vi "2D-LIF_CDN.vi"() -> ()   [LabVIEW 2022 SP3]
uses:
  dyelaser.lib/Sirah Control API.llb/SC API Burst Scan Mode.ctl
panel:
  out "Final.Gate.Delay":u64=600
  in  "New Scan":bool
  in  "Shut Down":bool
  out "ScanWhat?":enum16{"Nothing", "Lumonics", "Delay"}(ring)
  in  "Pause Scan":bool
  in  "Live Monitor":bool
  in  "force continue":bool
  in  "Force stop":bool
  out "State":T1(ring)=enum."Wait for input"
  in  "Abort Scan":bool
  in  "Camera":T2={"Gate.Delay"=0, "Delay.Step"=0, "Gate.Duration"=50, "#Accum"=30, "SetpointTemp"=-30, "Last Temp"=0, "Current Temp"=0}
  out "Data":cluster{"CCD":i32[], "2D LIF data":i32[][]}
  in  "Mono":T3={"Offset (cm-1)"=200.0, "Step (cm-1)"=2.0, "Counter"=165.13, "Scan Step/Mono Step"=1, "Status"={"Moving"=FALSE, "Home"=FALSE, "Hi"=FALSE, "Low"=FALSE}, "nm"=660.502, "Mono port"="McPherson"} {"nm" format="%.3f"; "Scan Step/Mono Step" format="%.2f"; "Counter" format="%.2g"; "Step (cm-1)" format="%.1f"; "Offset (cm-1)" format="%#.4g"}
  in  "DyeLaser":T4={"Scan.Start (cm-1)"=15340.0, "Scan.Stop (cm-1)"=15365.0, "Scan.step (cm-1)"=0.05, "Dye laser port"="USB0::0x17E7::0x0500::11-20-16::INSTR", "Laser"=enum."Hyperdye", "NPoints"=501, "CurrentStep"=0, "Current.cm-1"=15340.0} {"Current.cm-1" format="%.2f"; "Scan.Stop (cm-1)" format="%.2f"; "Scan.step (cm-1)" format="%.2g"; "Scan.Start (cm-1)" format="%.2f"}
  # "ns"
  # "ns"
  # "ns"
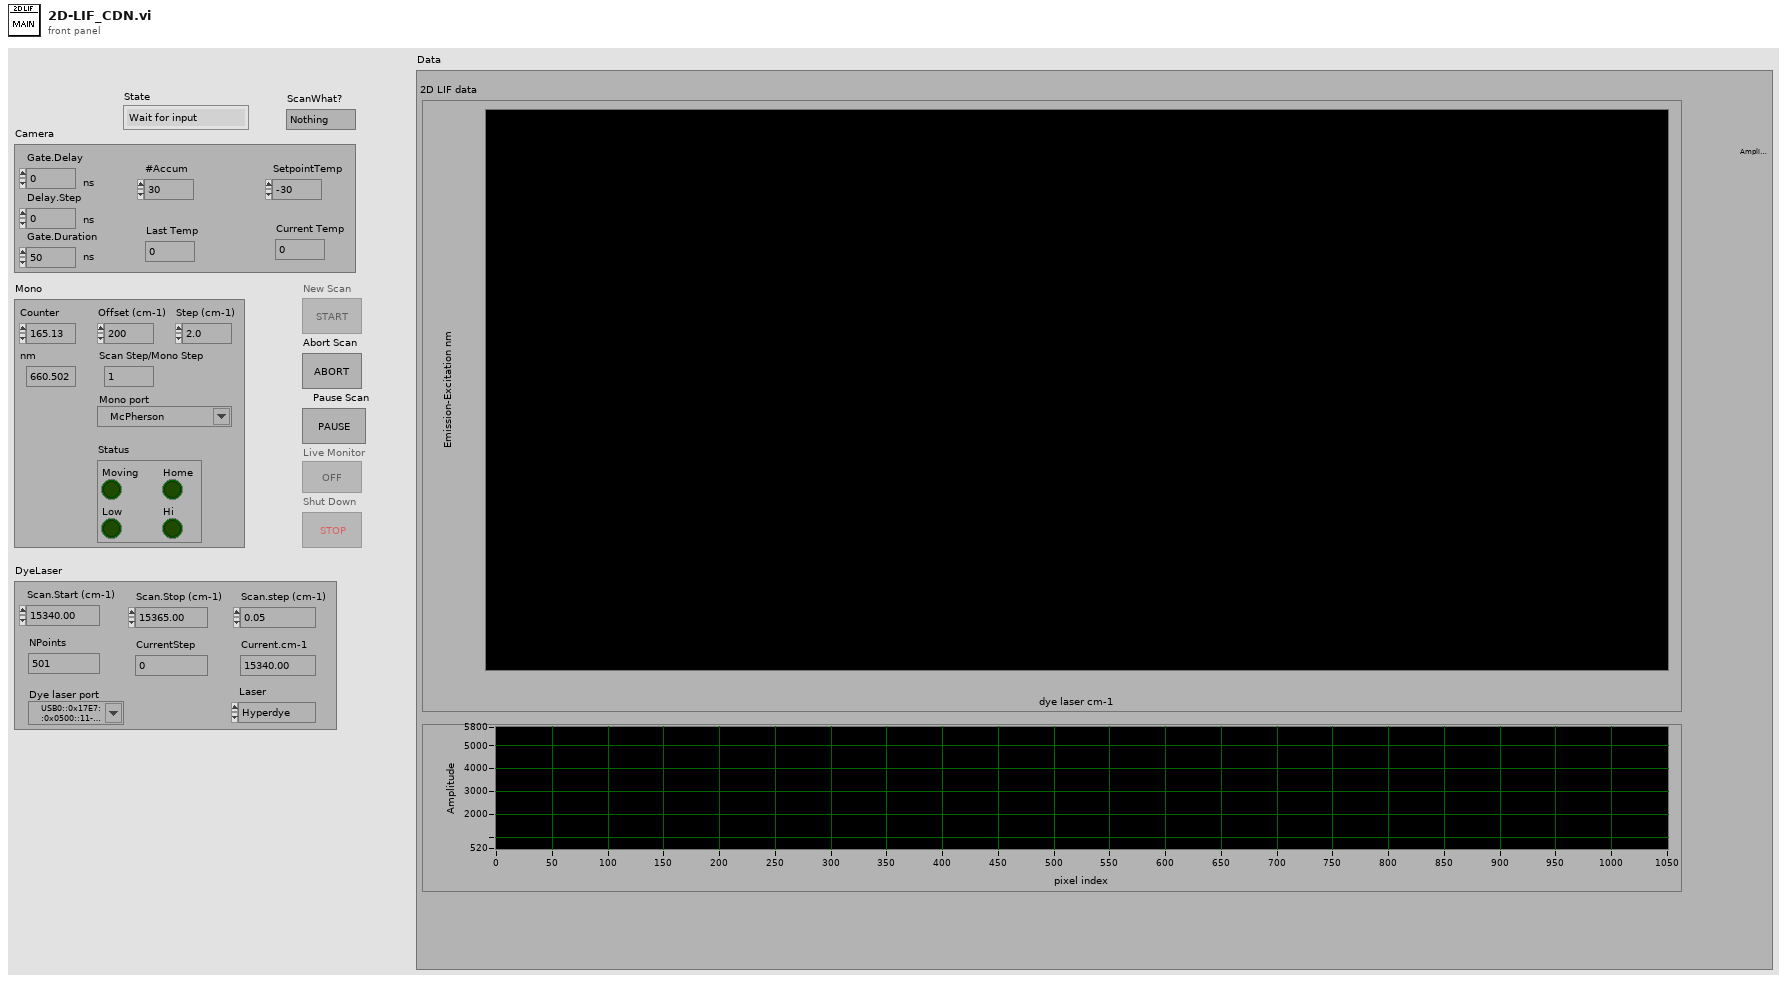
[diagram p1: front panel]
types:
  T1 = enum16{"Connect", "Wait for input", "Initialize", "Live", "Start Scan", "Continue Scan", "End Scan", "Shut Down"}
  T2 = cluster{"Gate.Delay":u64, "Delay.Step":u64, "Gate.Duration":u64, "#Accum":i32, "SetpointTemp":i32, "Last Temp":i32, "Current Temp":i32}
  T3 = cluster{"Offset (cm-1)":dbl, "Step (cm-1)":dbl, "Counter":dbl, "Scan Step/Mono Step":i32, "Status":cluster{"Moving":bool, "Home":bool, "Hi":bool, "Low":bool}, "nm":dbl, "Mono port":refnum<visa-resource-name>}
  T4 = cluster{"Scan.Start (cm-1)":dbl, "Scan.Stop (cm-1)":dbl, "Scan.step (cm-1)":dbl, "Dye laser port":refnum<visa-resource-name>, "Laser":enum16{"Syrah", "Hyperdye"}, "NPoints":i32, "CurrentStep":i32, "Current.cm-1":dbl}
  T5 = typedef "SC API Burst Scan Mode.ctl" = enum16{"Wavelength (nm), use increment", "Wavenumber (cm-1), use increment", "Frequency (Hz), use increment", "x", "xx", "xxx", "xxxx", "xxxxx", "xxxxxx", "xxxxxxx", "Wavelength (nm), use number", "Wavenumber (cm-1), use number", "Frequency (Hz), use number"}
  T6 = enum8{"Enabled", "Disabled", "Disabled and Grayed Out"}
  T7 = cluster{"offset (cm-1)":dbl, "step (cm-1)":dbl, "Counter":dbl, "Scanstep/monostep":i32, "Status":cluster{"Moving":bool, "Home":bool, "Hi":bool, "Low":bool}, "nm":dbl, "mono port":refnum<visa-resource-name>}
  T8 = cluster{"Scan.Start (cm-1)":dbl, "Scan.Stop (cm-1)":dbl, "Scan.step (cm-1)":dbl, "dye laser port":refnum<visa-resource-name>, "Laser":enum16{"Syrah", "Hyperdye"}, "NSteps":i32, "CurrentStep":i32, "Current.cm-1":dbl}
  T9 = cluster{"offset (cm-1)":dbl, "step (cm-1)":dbl, "Counter":dbl, "Scanstep/monostep":i32, "Status":cluster{"Moving":bool, "Home":bool, "Hi":bool, "Low":bool}, "nm":dbl, "Mono port":refnum<visa-resource-name>}
  T10 = cluster{"Scan.Start (cm-1)":dbl, "Scan.Stop (cm-1)":dbl, "Scan.step (cm-1)":dbl, "dye laser port":refnum<visa-resource-name>, "Laser":enum16{"Syrah", "Hyperdye"}, "NPoints":i32, "CurrentStep":i32, "Current.cm-1":dbl}
  T11 = cluster{"offset (cm-1)":dbl, "step (cm-1)":dbl, "Counter":dbl, "Scanstep/monostep":i32, "Status":cluster{"Moving":bool, "Home":bool, "Hi":bool, "Low":bool}, "nm":dbl, "VISA resource name":refnum<visa-resource-name>}
  T12 = cluster{"Scan.Start (cm-1)":dbl, "Scan.Stop (cm-1)":dbl, "Scan.step (cm-1)":dbl, "VISA resource name":refnum<visa-resource-name>, "Laser":enum16{"Syrah", "Hyperdye"}, "NSteps":i32, "CurrentStep":i32, "Current.cm-1":dbl}
  T13 = cluster{"Scan.Start (cm-1)":dbl, "Scan.Stop (cm-1)":dbl, "Scan.step (cm-1)":dbl, "Dye laser port":refnum<visa-resource-name>, "Laser":enum16{"Syrah", "Hyperdye"}, "NSteps":i32, "CurrentStep":i32, "Current.cm-1":dbl}
  T14 = typedef "LVRangeTypeDef.ctl" = cluster{"Minimum":dbl, "Maximum":dbl, "Increment":dbl, "Minor Increment":dbl, "Start":dbl}
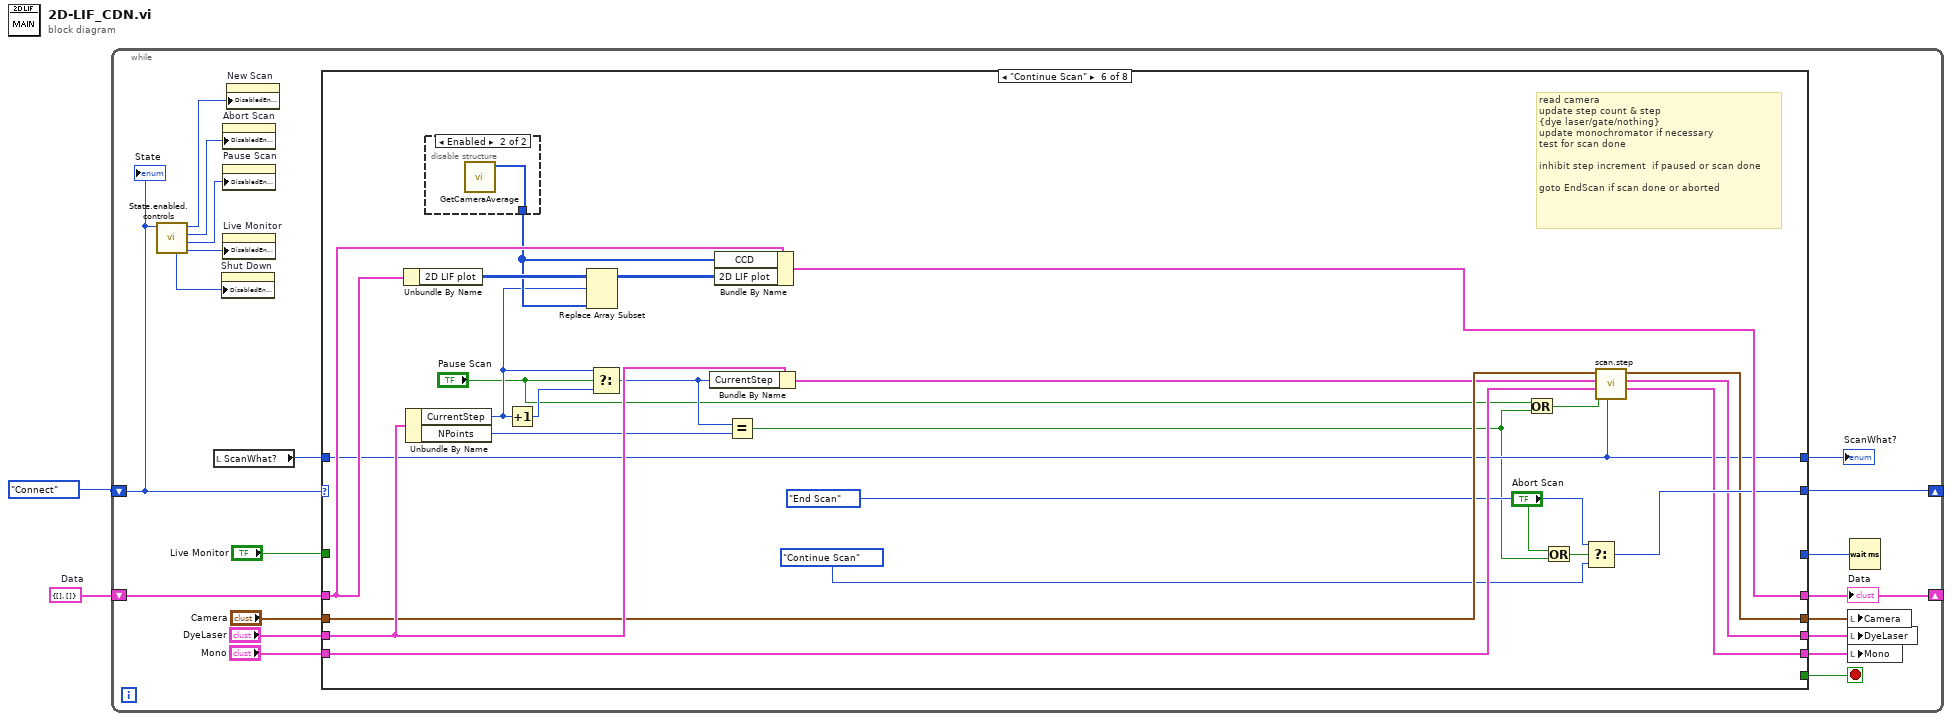
[diagram p0: block diagram]
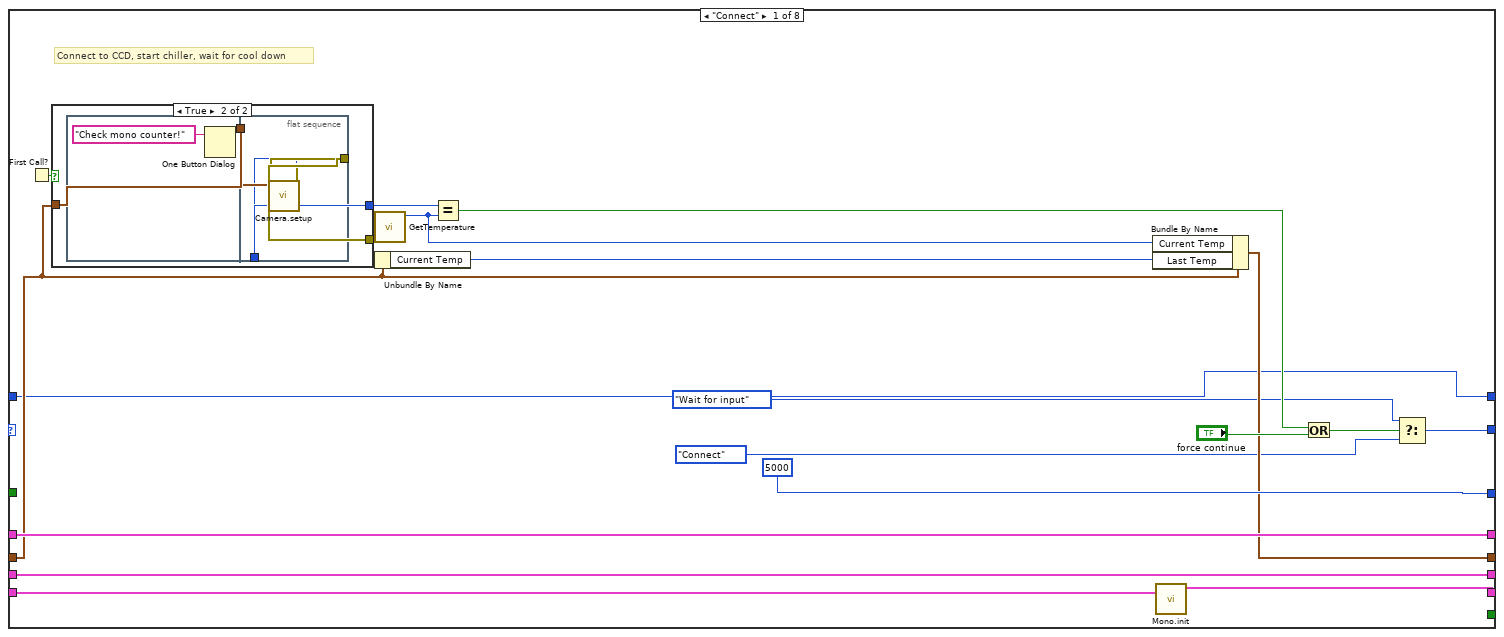
[diagram p2: hidden frame]
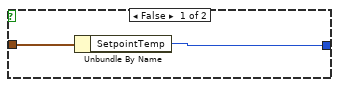
[diagram p3: hidden frame]
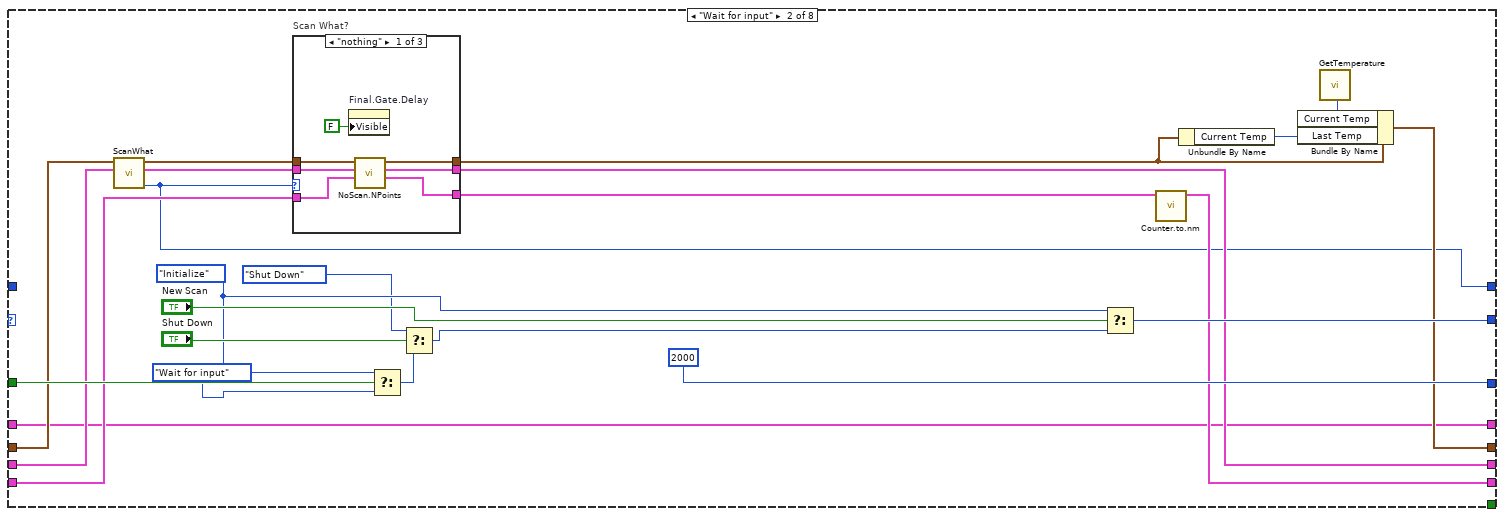
[diagram p4: hidden frame]
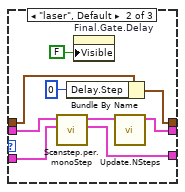
[diagram p5: hidden frame]
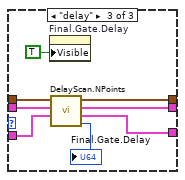
[diagram p6: hidden frame]
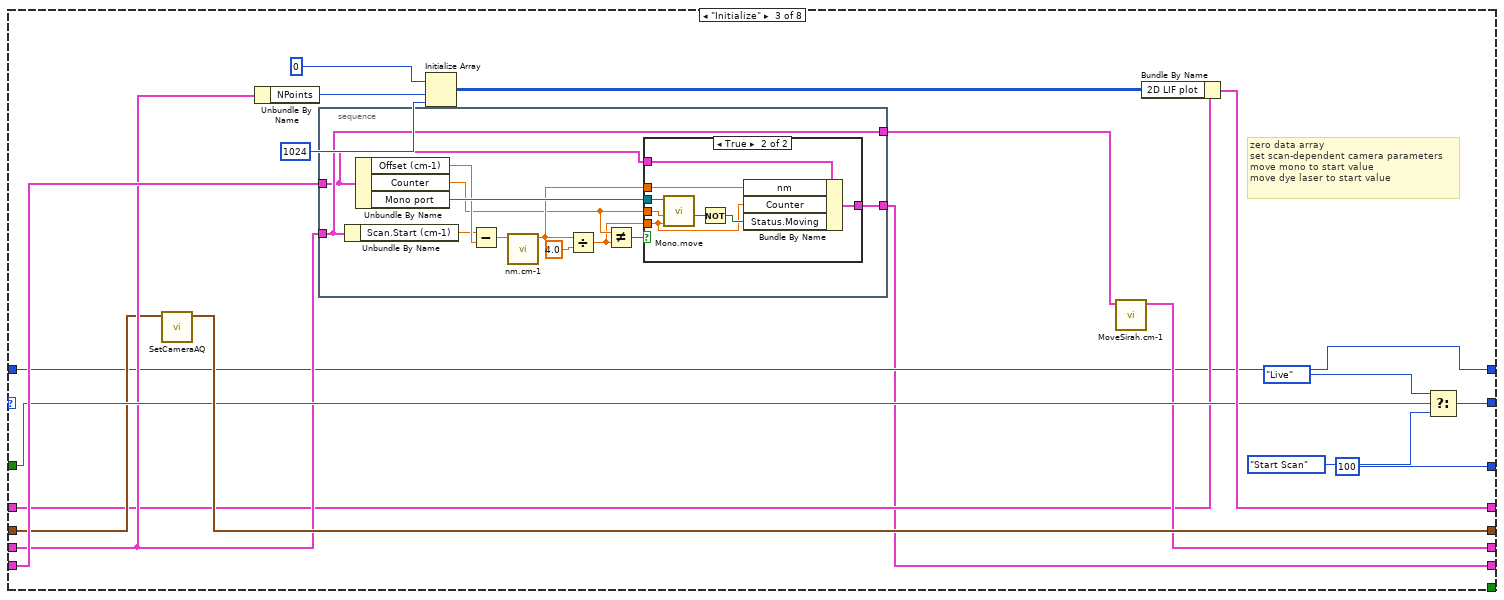
[diagram p7: hidden frame]
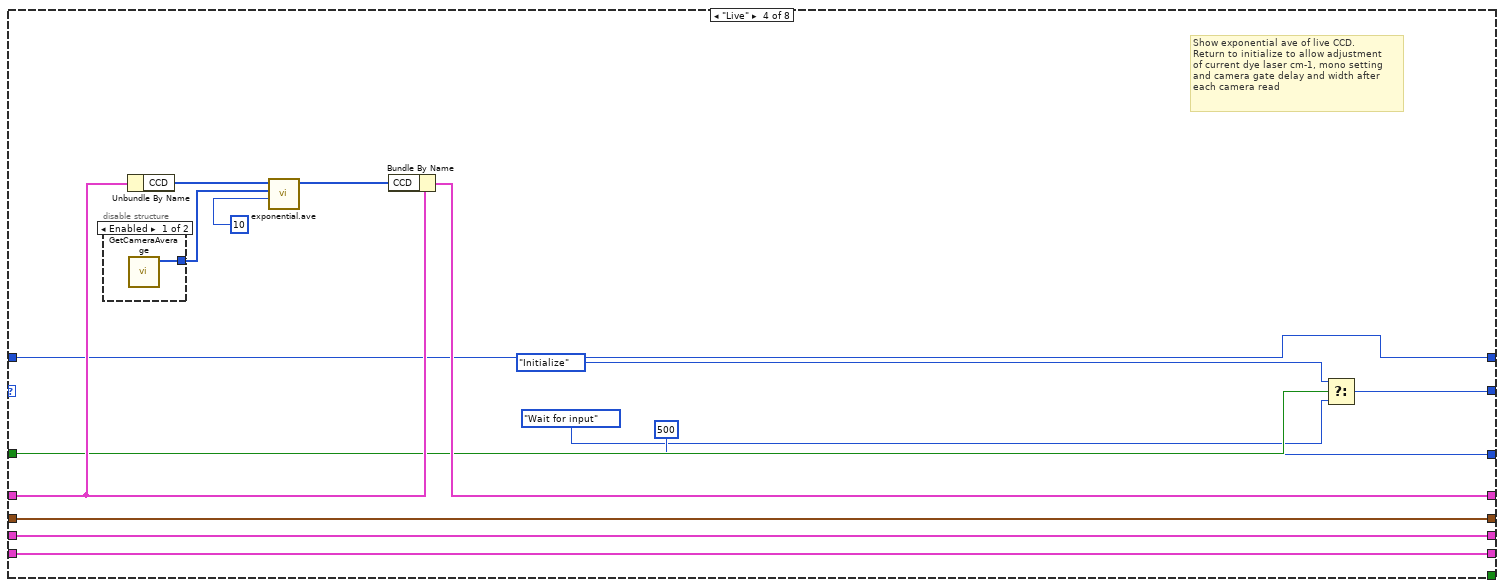
[diagram p9: hidden frame]
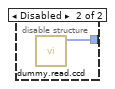
[diagram p10: hidden frame]
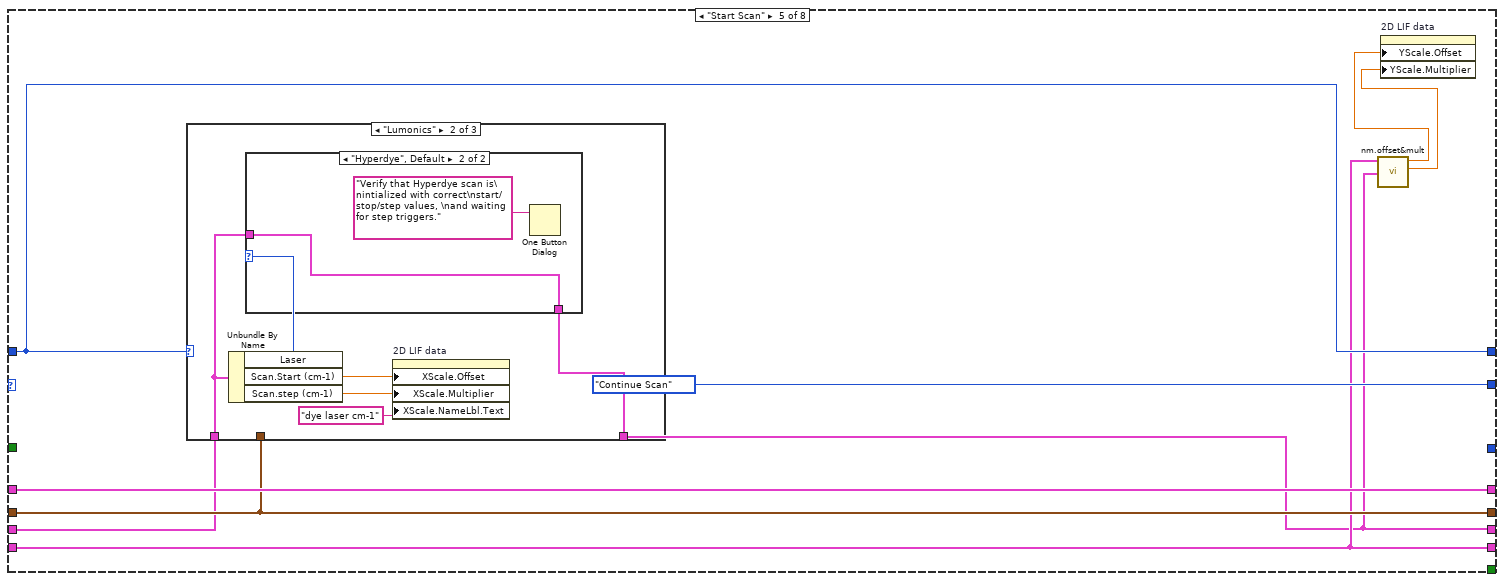
[diagram p11: hidden frame]
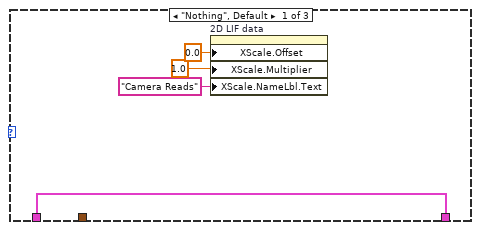
[diagram p12: hidden frame]
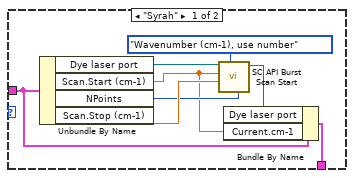
[diagram p13: hidden frame]
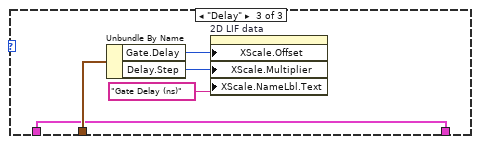
[diagram p14: hidden frame]
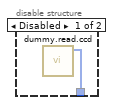
[diagram p15: hidden frame]
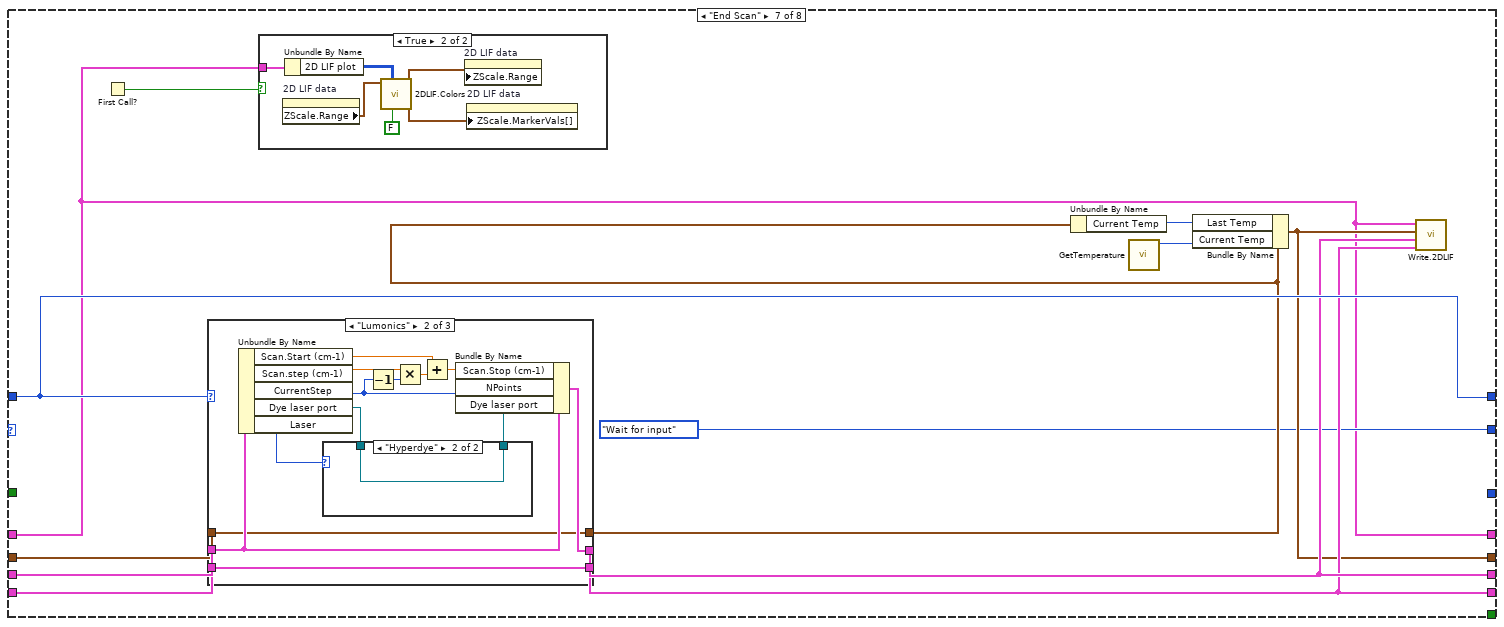
[diagram p16: hidden frame]
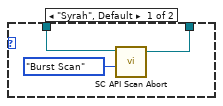
[diagram p19: hidden frame]
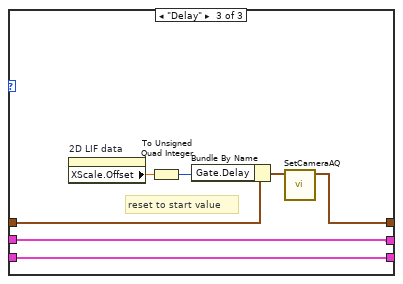
[diagram p20: hidden frame]
diagram:
  w2 = cluster{"CCD":i32[], "2D LIF plot":i32[][]} {"CCD"=[], "2D LIF plot"=[]}  # Data
  n1 = while {
    shift-right: [w20] -> _
    shift-left: w2 -> [w21]
    shift-right: [w6] -> _
    shift-left: T1."Connect" ("State") -> [w3]
    stop <- w22 stop-if-true
    n2 = call "State.enabled.controls.vi"("state"=w3) -> ("live"=w12:T6, "pause"=w11:T6, "abort"=w10:T6, "start"=w5:T6, "stop"=w4:T6)  [unwired: 6 in]
    n3 = local read "ScanWhat?"() -> (w9:enum16{"Nothing", "Lumonics", "Delay"})
    n4 = property on="Shut Down" class="Bool"("DisabledEnum"=w4) -> ()  [unwired: 2 in, 2 out]
    n5 = property on="Abort Scan" class="Bool"("DisabledEnum"=w10) -> ()  [unwired: 2 in, 2 out]
    n6 = property on="Pause Scan" class="Bool (strict)"("DisabledEnum"=w11) -> ()  [unwired: 2 in, 2 out]
    n7 = property on="Live Monitor" class="Bool (strict)"("DisabledEnum"=w12) -> ()  [unwired: 2 in, 2 out]
    n8 = property on="New Scan" class="Bool"("DisabledEnum"=w5) -> ()  [unwired: 2 in, 2 out]
    n9 = case shown="\"Continue Scan\"" w3 {
      tunnel: [_ _ _ _ _ _ _ w265] -> w22
      tunnel: w21 -> [w41 w52 w104 w152 w164 w214 w218 w274]
      tunnel: [w41 w52 w115 w150 w164 w209 w218 w274] -> w20
      tunnel: [w31 w56 w107 w147 w158 w201 w226 w267] -> w19
      tunnel: "Camera" -> [w26 w64 w105 w144 w163 w203 w222 w269]
      tunnel: [w32 w59 w112 w144 w163 w202 w220 w268] -> w13
      tunnel: "DyeLaser" -> [w31 w63 w106 w147 w162 w207 w225 w267]
      tunnel: "Mono" -> [w28 w65 w111 w151 w159 w198 w224 w270]
      tunnel: [u32 5000 u32 2000 ("milliseconds to wait") u32 100 ("milliseconds to wait") u32 500 ("milliseconds to wait") _ _ _ u32 5000] -> w16
      tunnel: [w27 w57 w99 w151 w159 w200 w223 w270] -> w15
      tunnel: [w29 w70 w110 w153 T1."Continue Scan" ("State") w206 T1."Wait for input" ("State") T1."Shut Down" ("State")] -> w6
      tunnel: "Live Monitor" -> [_ w68 w109 w148 _ _ _ _]
      tunnel: [w25 w51 w103 w142 w160 w197 w227 w264] -> w8
      tunnel: w9 -> [w25 _ w103 w142 w160 w197 w227 w264]
      frame "Connect" {
        # "Connect to CCD, start chiller, wait for cool down"
        n10 = First Call?() -> (First Call?: T/F=w40:bool)
        n11 = case shown="True" w40 {
          tunnel: [_ w45] -> w39
          tunnel: [w43 w44] -> w38
          tunnel: w26 -> [w42 w46]
          frame False {
            n12 = Unbundle By Name(w42) -> ("SetpointTemp"=w43:i32)
          }
          frame True {
            n13 = flat-sequence {
              tunnel: w46 -> [w50]
              tunnel: [w49] -> w45
              tunnel: [w48] -> w44
              frame #0 {
                n14 = One Button Dialog(message="Check mono counter!") -> ()  [unwired: 1 in, 1 out]
              }
              frame #1 {
                n15 = call "Camera.setup.vi"("Camera"=w50) -> ("error out"=w49:errorcluster, "SetpointTemp"=w48:i32)  [unwired: 8 in, 1 out]
              }
            }
          }
        }
        n16 = call "GetTemperature.vi"("error in (no error)"=w39) -> ("temperature"=w37:i32)  [unwired: 3 in, 3 out]
        n17 = Unbundle By Name(w26) -> ("Current Temp"=w30:i32)
        n18 = Equal?(x=w38, y=w37) -> (x = y?=w34:bool)
        n19 = Bundle By Name(cluster=w26, "Current Temp"=w37, "Last Temp"=w30) -> (w32:T2)
        n20 = call "Mono.init.vi"("Mono in"=w28) -> ("Mono out"=w27:T7)  [unwired: 10 in]
        n21 = Or(x=w34, y="force continue") -> (x .or. y?=w36:bool)
        n22 = Select(t=T1."Wait for input" ("State"), s=w36, f=T1."Connect" ("State")) -> (s? t:f=w29:T1)
      }
      frame "Wait for input" {
        w54 = T1."Initialize" ("State")
        n23 = call "ScanWhat.vi"("DyeLaser"=w63, "Camera"=w64) -> ("ScanWhat?"=w51:enum16{"nothing", "laser", "delay"}, "DyeLaser out"=w61:T8, "Camera out"=w62:T2)  [unwired: 7 in]
        n24 = case "Scan What?" shown="\"nothing\"" w51 {
          tunnel: w61 -> [w80 w89 w98]
          tunnel: w62 -> [w81 w83 w94]
          tunnel: w65 -> [w79 w90 w97]
          tunnel: [w78 w84 w93] -> w60
          tunnel: [w77 w86 w96] -> w56
          tunnel: [w76 w88 w95] -> w58
          frame "nothing" {
            n25 = property on="Final.Gate.Delay" class="DigNum (strict)"("Visible"=FALSE) -> ()  [unwired: 2 in, 2 out]
            n26 = call "NoScan.NPoints.vi"("Mono"=w79, "DyeLaser In"=w80, "Camera"=w81) -> ("Mono out"=w76:T9, "DyeLaser out"=w77:T10, "Camera out"=w78:T2)  [unwired: 6 in]
          }
          frame "laser", Default {
            n27 = call "Scanstep.per.monoStep.vi"("Mono in"=w90, "DyeLaser"=w89) -> ("Mono out"=w88:T11, "DyeLaser out"=w87:T12)  [unwired: 8 in]
            n28 = Bundle By Name(cluster=w83, "Delay.Step"=u64 0) -> (w84:T2)
            n29 = property on="Final.Gate.Delay" class="DigNum (strict)"("Visible"=FALSE) -> ()  [unwired: 2 in, 2 out]
            n30 = call "Update.NSteps.vi"("DyeLaser In"=w87) -> ("DyeLaser out"=w86:T10)  [unwired: 10 in]
          }
          frame "delay" {
            n31 = property on="Final.Gate.Delay" class="DigNum (strict)"("Visible"=TRUE) -> ()  [unwired: 2 in, 2 out]
            n32 = call "DelayScan.NPoints.vi"("Mono"=w97, "DyeLaser In"=w98, "Camera"=w94) -> ("Final.Gate.Delay"=→"Final.Gate.Delay":u64, "Mono out"=w95:T9, "DyeLaser out"=w96:T10, "Camera out"=w93:T2)  [unwired: 5 in]
          }
        }
        n33 = Select(t=w54, s=w68, f=T1."Wait for input" ("State")) -> (s? t:f=w69:T1)
        n34 = Select(t=T1."Shut Down" ("State"), s="Shut Down", f=w69) -> (s? t:f=w72:T1)
        n35 = Select(t=w54, s="New Scan", f=w72) -> (s? t:f=w70:T1)
        n36 = call "Counter.to.nm.vi"("Mono in"=w58) -> ("Mono out"=w57:T11)  [unwired: 10 in]
        n37 = Unbundle By Name(w60) -> ("Current Temp"=w66:i32)
        n38 = call "GetTemperature.vi"() -> ("temperature"=w67:i32)  [unwired: 4 in, 3 out]
        n39 = Bundle By Name(cluster=w60, "Current Temp"=w67, "Last Temp"=w66) -> (w59:T2)
      }
      frame "Initialize" {
        # "zero data array\nset scan-dependent camera parameters\nmove mono to start value\nmove dye laser to start value"
        n40 = call "SetCameraAQ.vi"("Camera"=w105) -> ("Camera out"=w112:T2)  [unwired: 9 in, 1 out]
        n41 = Unbundle By Name(w106) -> ("NPoints"=w113:i32)
        n42 = stacked-sequence {
          tunnel: w106 -> [w128]
          tunnel: [w128] -> w108
          tunnel: w111 -> [w127]
          tunnel: [w129] -> w99
          frame #0 {
            n43 = Unbundle By Name(w128) -> ("Scan.Start (cm-1)"=w124:dbl)
            n44 = Unbundle By Name(w127) -> ("Offset (cm-1)"=w125:dbl, "Counter"=w120:dbl, "Mono port"=w126:refnum<visa-resource-name>)
            n45 = Subtract(x=w124, y=w125) -> (x-y=w123:dbl)
            n46 = call "nm.cm-1.vi"("nm or cm-1 in"=w123) -> ("cm-1 or nm  out"=w122:dbl)  [unwired: 10 in]
            n47 = Divide(x=w122, y=4.0) -> (x/y=w119:dbl)
            n48 = Not Equal?(x=w120, y=w119) -> (x != y?=w118:bool)
            n49 = case shown="True" w118 {
              tunnel: w127 -> [w130 w137]
              tunnel: [w130 w138] -> w129
              tunnel: w120 -> [_ w134]
              tunnel: w126 -> [_ w133]
              tunnel: w122 -> [_ w132]
              tunnel: w119 -> [_ w131]
              frame False {
              }
              frame True {
                n50 = call "Mono.move.vi"("Target position"=w131, "Current position"=w134, "VISA resource name"=w133) -> ("done"=w136:bool)  [unwired: 8 in]
                n51 = Not(x=w136) -> (.not. x?=w135:bool)
                n52 = Bundle By Name(cluster=w137, "nm"=w132, "Counter"=w131, "Status.Moving"=w135) -> (w138:T3)
              }
            }
          }
        }
        n53 = Initialize Array(0 ("element"), w113, 1024 ("dimension size")) -> (w114:i32[][])
        n54 = call "MoveSirah.cm-1.vi"("DyeLaser"=w108) -> ("output cluster"=w107:T13)  [unwired: 10 in]
        n55 = Bundle By Name(cluster=w104, "2D LIF plot"=w114) -> (w115:cluster{"CCD":i32[], "2D LIF plot":i32[][]})
        n56 = Select(t=T1."Live" ("State"), s=w109, f=T1."Start Scan" ("State")) -> (s? t:f=w110:T1)
      }
      frame "Live" {
        # "Show exponential ave of live CCD.\nReturn to initialize to allow adjustment\nof current dye laser cm-1, mono setting\nand camera gate delay and width after \neach camera read"
        n57 = disable-structure shown="Enabled" {
          disable-tunnel: [w154 w155] -> w149
          frame Enabled {
            n58 = call "GetCameraAverage.vi"() -> ("data"=w154:i32[])  [unwired: 10 in, 1 out]
          }
          frame Disabled {
            n59 = call "dummy.read.ccd.vi"() -> ("Array"=w155:i32[])  [unwired: 11 in]
          }
        }
        n60 = Unbundle By Name(w152) -> ("CCD"=w146:i32[])
        n61 = call "exponential.ave.vi"("continuous ave"=10, "Array in"=w149, "CCD"=w146) -> ("Array out"=w145:i32[])  [unwired: 8 in]
        n62 = Bundle By Name(cluster=w152, "CCD"=w145) -> (w150:cluster{"CCD":i32[], "2D LIF plot":i32[][]})
        n63 = Select(t=T1."Initialize" ("State"), s=w148, f=T1."Wait for input" ("State")) -> (s? t:f=w153:T1)
      }
      frame "Start Scan" {
        n64 = case shown="\"Lumonics\"" w160 {
          tunnel: [w165 w169 w185] -> w158
          tunnel: w162 -> [w165 w173 w185]
          tunnel: w163 -> [_ _ w189]
          frame "Nothing", Default {
            n65 = property on="2D LIF data" class="IntGraph (strict)"("XScale.Offset"=0.0 ("X Scale.Offset and Multiplier:Offset"), "XScale.Multiplier"=1.0 ("X Scale.Offset and Multiplier:Multiplier"), "XScale.NameLbl.Text"="Camera Reads" ("X Scale.Name Label.Text")) -> ()  [unwired: 2 in, 2 out]
          }
          frame "Lumonics" {
            n66 = Unbundle By Name(w173) -> ("Laser"=w174:enum16{"Syrah", "Hyperdye"}, "Scan.Start (cm-1)"=w170:dbl, "Scan.step (cm-1)"=w172:dbl)
            n67 = case shown="\"Hyperdye\", Default" w174 {
              tunnel: w173 -> [w177 w183]
              tunnel: [w178 w183] -> w169
              frame "Syrah" {
                n68 = Unbundle By Name(w177) -> ("Dye laser port"=w181:refnum<visa-resource-name>, "Scan.Start (cm-1)"=w176:dbl, "NPoints"=w179:i32, "Scan.Stop (cm-1)"=w180:dbl)
                n69 = call "SC API Burst Scan Start.vi"("Number of pos (10)"=w179, "Burst Speed Scan Mode (Wavelength, increment)"=SC_API_Burst_Scan_Mode."Wavenumber (cm-1), use number", "Scan To"=w180, "Scan From"=w176, "VISA Resource Name"=w181) -> ("VISA Resource Name Out"=w175:refnum<visa-resource-name>)  [unwired: 5 in, 1 out]
                n70 = Bundle By Name(cluster=w177, "Dye laser port"=w175, "Current.cm-1"=w176) -> (w178:T4)
              }
              frame "Hyperdye", Default {
                n71 = One Button Dialog(message="Verify that Hyperdye scan is\nintialized with correct\nstart/stop/step values, \nand waiting for step triggers.") -> ()  [unwired: 1 in, 1 out]
              }
            }
            n72 = property on="2D LIF data" class="IntGraph (strict)"("XScale.Offset"=w170, "XScale.Multiplier"=w172, "XScale.NameLbl.Text"="dye laser cm-1" ("X Scale.Name Label.Text")) -> ()  [unwired: 2 in, 2 out]
          }
          frame "Delay" {
            n73 = Unbundle By Name(w189) -> ("Gate.Delay"=w188:u64, "Delay.Step"=w187:u64)
            n74 = property on="2D LIF data" class="IntGraph (strict)"("XScale.Offset"=w188, "XScale.Multiplier"=w187, "XScale.NameLbl.Text"="Gate Delay (ns)" ("X Scale.Name Label.Text")) -> ()  [unwired: 2 in, 2 out]
          }
        }
        n75 = call "nm.offset&mult.vi"("DyeLaser"=w158, "Mono"=w159) -> ("y multiplier (nm/pixel)"=w157:dbl, "y offset (nm)"=w156:dbl)  [unwired: 8 in]
        n76 = property on="2D LIF data" class="IntGraph (strict)"("YScale.Offset"=w156, "YScale.Multiplier"=w157) -> ()  [unwired: 2 in, 2 out]
      }
      frame "Continue Scan" {
        # "read camera\nupdate step count & step \n{dye laser/gate/nothing}\nupdate monochromator if necessary\ntest for scan done\n\ninhibit step increment  if paused or scan done\n\ngoto EndScan if scan done or aborted"
        n77 = Unbundle By Name(w214) -> ("2D LIF plot"=w213:i32[][])
        n78 = Unbundle By Name(w207) -> ("CurrentStep"=w195:i32, "NPoints"=w205:i32)
        n79 = disable-structure shown="Enabled" {
          disable-tunnel: [w215 w216] -> w208
          frame Disabled {
            n80 = call "dummy.read.ccd.vi"() -> ("Array"=w215:i32[])  [unwired: 11 in]
          }
          frame Enabled {
            n81 = call "GetCameraAverage.vi"() -> ("data"=w216:i32[])  [unwired: 10 in, 1 out]
          }
        }
        n82 = Increment(x=w195) -> (x+1=w196:i32)
        n83 = Replace Array Subset(array=w213, new element=w208, index (row)=w195) -> (w212:i32[][])  [unwired: 1 in]
        n84 = Select(t=w195, s="Pause Scan", f=w196) -> (s? t:f=w194:i32)
        n85 = Bundle By Name(cluster=w207, "CurrentStep"=w194) -> (w199:T4)
        n86 = Bundle By Name(cluster=w214, "CCD"=w208, "2D LIF plot"=w212) -> (w209:cluster{"CCD":i32[], "2D LIF plot":i32[][]})
        n87 = Equal?(x=w194, y=w205) -> (x = y?=w190:bool)
        n88 = Or(x="Pause Scan", y=w190) -> (x .or. y?=w204:bool)
        n89 = Or(x="Abort Scan", y=w190) -> (x .or. y?=w211:bool)
        n90 = Select(t=T1."End Scan" ("State"), s=w211, f=T1."Continue Scan" ("State")) -> (s? t:f=w206:T1)
        n91 = call "scan.step.vi"("ScanWhat?"=w197, "inhibit\nstep"=w204, "Mono"=w198, "DyeLaser"=w199, "Camera"=w203) -> ("Mono.out"=w200:T7, "DyeLaser out"=w201:T8, "Camera out"=w202:T2)  [unwired: 4 in]
      }
      frame "End Scan" {
        n92 = First Call?() -> (First Call?: T/F=w217:bool)
        n93 = case shown="\"Lumonics\"" w227 {
          tunnel: w225 -> [w237 w243 w261]
          tunnel: [w237 w244 w261] -> w226
          tunnel: w224 -> [w236 w242 w262]
          tunnel: [w236 w242 w262] -> w223
          tunnel: w222 -> [w238 w240 w260]
          tunnel: [w238 w240 w256] -> w221
          frame "Nothing", Default {
            # "probably nothing needs doing here"
          }
          frame "Lumonics" {
            n94 = Unbundle By Name(w243) -> ("Scan.Start (cm-1)"=w247:dbl, "Scan.step (cm-1)"=w245:dbl, "CurrentStep"=w249:i32, "Dye laser port"=w250:refnum<visa-resource-name>, "Laser"=w241:enum16{"Syrah", "Hyperdye"})
            n95 = case shown="\"Hyperdye\"" w241 {
              tunnel: [w254 w255] -> w251
              tunnel: w250 -> [w253 w255]
              frame "Syrah", Default {
                n96 = call "SC API Scan Abort.vi"("Scan Method (CSS)"=enum16{"Constant Speed Scan", "Burst Scan"}."Burst Scan", "VISA Resource Name"=w253) -> ("VISA Resource Name Out"=w254:refnum<visa-resource-name>)  [unwired: 8 in, 1 out]
              }
              frame "Hyperdye" {
              }
            }
            n97 = Decrement(x=w249) -> (x-1=w239:i32)
            n98 = Multiply(x=w245, y=w239) -> (x*y=w246:dbl)
            n99 = Add(x=w247, y=w246) -> (x+y=w248:dbl)
            n100 = Bundle By Name(cluster=w243, "Scan.Stop (cm-1)"=w248, "NPoints"=w249, "Dye laser port"=w251) -> (w244:T4)
          }
          frame "Delay" {
            # "reset to start value"
            n101 = property on="2D LIF data" class="IntGraph (strict)"() -> ("XScale.Offset"=w259:dbl)  [unwired: 2 in, 2 out]
            n102 = To Unsigned Quad Integer(1:w259) -> (0:w258:u64)
            n103 = Bundle By Name(cluster=w260, "Gate.Delay"=w258) -> (w257:T2)
            n104 = call "SetCameraAQ.vi"("Camera"=w257) -> ("Camera out"=w256:T2)  [unwired: 9 in, 1 out]
          }
        }
        n105 = case shown="True" w217 {
          tunnel: w218 -> [_ w230]
          frame False {
          }
          frame True {
            n106 = property on="2D LIF data" class="IntGraph (strict)"() -> ("ZScale.Range"=w234:T14)  [unwired: 2 in, 2 out]
            n107 = Unbundle By Name(w230) -> ("2D LIF plot"=w232:i32[][])
            n108 = call "2DLIF.Colors.vi"("override scale?"=FALSE, "Intensity Graph"=w232, "ZScale.Range in"=w234) -> ("Zscale.MarkerVals[]"=w235:cluster{dbl, u32}[], "ZScale.Range out"=w233:T14)  [unwired: 6 in, 1 out]
            n109 = property on="2D LIF data" class="IntGraph (strict)"("ZScale.Range"=w233) -> ()  [unwired: 2 in, 2 out]
            n110 = property on="2D LIF data" class="IntGraph (strict)"("ZScale.MarkerVals[]"=w235) -> ()  [unwired: 2 in, 2 out]
          }
        }
        n111 = Unbundle By Name(w221) -> ("Current Temp"=w228:i32)
        n112 = call "GetTemperature.vi"() -> ("temperature"=w229:i32)  [unwired: 4 in, 3 out]
        n113 = Bundle By Name(cluster=w221, "Last Temp"=w228, "Current Temp"=w229) -> (w220:T2)
        n114 = call "Write.2DLIF.vi"("Mono"=w223, "DyeLaser"=w226, "Camera"=w220, "Data"=w218) -> ()  [unwired: 7 in, 1 out]
      }
      frame "Shut Down" {
        # "turn off CCD chiller; wait for warmup,\nclose communication channels\nthen quit"
        n115 = First Call?() -> (First Call?: T/F=w273:bool)
        n116 = case shown="True" w273 {
          tunnel: [w275 _] -> w271
          tunnel: w267 -> [_ w282]
          tunnel: w270 -> [_ w281]
          tunnel: [w278 w280] -> w268
          tunnel: w269 -> [w276 w280]
          frame False {
            n117 = Unbundle By Name(w276) -> ("Current Temp"=w277:i32)
            n118 = call "GetTemperature.vi"() -> ("temperature"=w279:i32)  [unwired: 4 in, 3 out]
            n119 = Greater Than 0?(x=w279) -> (x > 0?=w275:bool)
            n120 = Bundle By Name(cluster=w276, "Last Temp"=w277, "Current Temp"=w279) -> (w278:T2)
            n121 = case shown="True" w275 {
              frame False {
              }
              frame True {
                n122 = call "ShutDown.vi"() -> ()  [unwired: 2 in, 2 out]
              }
            }
          }
          frame True {
            n123 = call "Close.mono.vi"("Mono"=w281) -> ()  [unwired: 11 in]
            n124 = call "Close.dyelaser.vi"("DyeLaser"=w282) -> ()  [unwired: 11 in]
            n125 = call "CoolerOFF.vi"() -> ()  [unwired: 2 in, 2 out]
          }
        }
        n126 = Or(x=w271, y="Force stop") -> (x .or. y?=w265:bool)
      }
    }
    "Data" <- w20
    "ScanWhat?" <- w8
    n127 = local write "Camera"(w13) -> ()
    n128 = local write "DyeLaser"(w19) -> ()
    n129 = local write "Mono"(w15) -> ()
    n130 = Wait (ms)(milliseconds to wait=w16) -> ()  [unwired: 1 out]
    "State" <- w3
  }
